vi "Sys config-process changes.vi"(11 "Initial Configuration":T1={"Triggers output setup"=[], "General trigger settings"={"Trigger 1 function"=enum."Line trigger", "Triggers loop clock (MHz)"=115.0}, "Calibration settings"={"Pockels cal.Zoom"=0, "Pockels cal.Dwell time (µs)"=0.0}, "Hardware Configuration"={"Dev. PC"=FALSE, "Swap XY on stage"=FALSE, "No of AOD"=0, "MC Supported"=FALSE, "Axial MC"=FALSE, "Computer MAC address"="", "Externalise Triggers"=FALSE, "Trigger HW config"={"Available Device List"=0, "Device Address"=""}, "DAQmx Chan"={"Pockels AO"="", "Hard shutter AO"="", "PMT AOs"="", "Galvo AOs"="", "Power meter AI"=""}, "XYZ Stage Control Config"=enum."None", "XY stage available"=FALSE, "XY Comms Config Cluster"={"Name"="", "Device Address"="", "Port "=0, "Baudrate"=0, "Comms Type"=enum."GPIB-IEEE488"}, "Y stage available"=FALSE, "Y Comms Config Cluster"={"Name"="", "Device Address"="", "Port "=0, "Baudrate"=0, "Comms Type"=enum."GPIB-IEEE488"}, "Z stage available"=FALSE, "Z Comms Config Cluster "={"Name"="", "Device Address"="", "Port "=0, "Baudrate"=0, "Comms Type"=enum."GPIB-IEEE488"}, "Encoder available"=FALSE, "Encoder"={"IP address"="224.0.1.103", "Port"=7000, "Wheel radius (cm)"=16.0, "Encoder Trigger"=""}, "VidRec available"=FALSE, "Cam VidRec"={"DO flag-Video record"="", "DO flag-Trial start"=""}, "Laser Power Control HW config"={"Laser Power Control"="", "Laser Power Modulation Control"=enum."NI"}, "Laser 1 available"=FALSE, "Laser 1 config cluster"={"COM port"="COM7", "Baud Rate"=0, "Type"=""}, "Prechirper 1 available"=FALSE, "Prechirper 1 config cluster"={"Type"="", "Baud Rate"=0, "COM port"="COM7"}, "Control system.FPGA available?"=FALSE, "Control Sys. HW config"={"Control system.FPGA Type"=enum."Virtex 5", "Control system.Network adapter name"="", "Control system.MAC address"="", "Control system.Ethernet Port"=0, "Control system.Ethernet Port Opened"=FALSE}, "DAQ FPGA HW Config"={"FGPA Ref"=refnum, "Target"="RIO0", "input card type"=enum."AC Card"}, "PMT Control Voltage Limits"={"Lower Limit"=0.0, "Upper Limit"=0.0}}, "System Config"={"Laser wavelength (nm)"=920.0, "DAQ FPGA System"={"Clock Freq (MHz) "=200.0, "Samples Wait after Trigger"=5080, "AOD fill"=4900, "StartupDelay"=0, "Slip Cycle (clock cycles)"=600000, "Add Cycle"=TRUE}, "Control system"={"AOD 1 Amplitude"=0, "AOD 2 Amplitude"=0, "AOD 3 Amplitude"=0, "AOD 4 Amplitude"=0, "AOD 5 Amplitude"=0, "AOD 6 Amplitude"=0, "T0 (ns)"=0.0, "Ta (ns)"=0.0, "Data Time Interval (ns)"=0.0, "Ctrl FPGA Clock (MHz)"=240.0}}, "Calibration config."={"Current Objective"="", "Objective Settings"=[], "PreChirper Values Preset ?"=FALSE, "PreChirper Settings"=[], "PreChirper Constants"={"a 1"=0, "b 1"=0, "c 1"=0, "a 2"=0, "b 2"=0, "c 2"=0, "lmin"=0, "lmax"=0}}, "General Setup"={"Microscope ID"="003", "Microscope Type"="AOLM", "Revision Number"="1.0.0.0", "Advanced Imaging"=FALSE, "Error Logging"=FALSE, "Performance Monitoring"=FALSE, "Max Allowed Trial Length"=60.0, "Initial Scan Resolution"=512.0, "Initial Acceptance Angle"=5.0, "Initial Laser Wavelength"=900.0, "Initial Dwell Time"=900.0}, "AOD Settings - distilled"={"AOD 1 thickness (mm)"=0.0, "AOD 2 thickness (mm)"=0.0, "AOD 3 thickness (mm)"=110.0, "AOD 4 thickness (mm)"=135.0, "AOD 1-2 separation (mm)"=15.0, "AOD 2-3 separation (mm)"=15.0, "AOD 3-4 separation (mm)"=15.0, "AOD 1 Centre (mm)"=15.0, "AOD 2 Centre (mm)"=50.0, "AOD 3 Centre (mm)"=50.0, "AOD 4 Centre (mm)"=50.0, "AOD 1 X Offset"=15.0, "AOD 2 X Offset"=1.0, "AOD 3 X Offset"=1.0, "AOD 4 X Offset"=1.0, "AOD 1 Y Offset"=1.0, "AOD 2 Y Offset"=1.0, "AOD 3 Y Offset"=1.0, "AOD 4 Y Offset"=1.0, "Timing Offset AOD 1"=0.0, "Timing Offset AOD 2"=0.0, "Timing Offset AOD 3"=0.0, "Timing Offset AOD 4"=0.0, "AOL centre wavelength (nm)"=1.0, "AOL centre frequency (MHz)"=1.0, "Pair deflection ratio"=1.0, "AOL aperture (mm)"=0.0, "AOD fill time (us)"=0.0, "Diffraction mode"=0.0, "Crystal length (mm)"=0.0, "Acoustic velocity (m/s)"=1.0, "AOD Ord. Refractive index"=20000.0}} {"System Config"."Control system"."Ctrl FPGA Clock (MHz)" min=80.0 max=500.0 step=1.0; "System Config"."Control system"."Data Time Interval (ns)" min=0.0 max=2048.0 step=1.0; "System Config"."Control system"."Ta (ns)" min=0.0 max=2048.0 step=1.0; "System Config"."Control system"."T0 (ns)" min=0.0 max=2048.0 step=1.0; "System Config"."Control system"."AOD 6 Amplitude" min=0 max=2048 step=1; "System Config"."Control system"."AOD 5 Amplitude" min=0 max=2048 step=1; "System Config"."Control system"."AOD 4 Amplitude" min=0 max=2048 step=1; "System Config"."Control system"."AOD 3 Amplitude" min=0 max=2048 step=1; "System Config"."Control system"."AOD 2 Amplitude" min=0 max=2048 step=1; "System Config"."Control system"."AOD 1 Amplitude" min=0 max=2048 step=1; "System Config"."Laser wavelength (nm)" min=800.0 max=1080.0 step=1.0; "Hardware Configuration"."Encoder"."Wheel radius (cm)" format="%#_13g"; "General trigger settings"."Triggers loop clock (MHz)" format="%#_13g"; "Triggers output setup"."Pulse width (us)" min=10 max=5000 step=1 format="%.0fµs"}) -> ()   [LabVIEW 2020]
uses:
  Visualisation/Functional Imaging Viewer/Typedefs/Get-Set-Clear Control.ctl
  Typedefs/HW config states enum.ctl
  Typedefs/Save-Load enum.ctl
  Peripherals Control/Triggers/Typedefs/Trigger setup element cluster.ctl
  Peripherals Control/Triggers/Typedefs/Triggers output setup.ctl
  Configuration code/Typedefs/Pockels Calibration settings cluster.ctl
  Typedefs/Trigger 1 selector enum.ctl
  Peripherals Control/Triggers/Typedefs/General trigger settings cluster.ctl
  Typedefs/Cam VidRec HW config setup cluster.ctl
  Typedefs/Control Sys HW config cluster.ctl
  <vilib>/userDefined/High Color/nirio_resource_hc.ctl
  Typedefs/FPGA input type AC-DC.ctl
  RIG-SPECIFIC FILES/FPGA Refs/FPGA Ref.ctl
  Typedefs/DAQ FPGA HW config cluster.ctl
  Typedefs/DAQmx physical channels cluster.ctl
  Typedefs/Encoder config cluster.ctl
  Typedefs/Laser 1 config cluster.ctl
  Typedefs/PreChirper 1 config cluster.ctl
  Typedefs/Laser Power Control HW config.ctl
  Typedefs/Triggers HW config.ctl
  Typedefs/Hardware Configuration settings.ctl
  Typedefs/DAQ FPGA system config.ctl
  Typedefs/CTRL system config.ctl
  Typedefs/System Configuration.ctl
  Typedefs/Objective Config.ctl
  Typedefs/Prechirper Cal Config.ctl
  Typedefs/PreChirper constants.ctl
  Typedefs/Calibration config.ctl
  Typedefs/General Setup.ctl
  Typedefs/AOD Settings-distilled.ctl
  Configuration code/Typedefs/Initial config.ctl
  Typedefs/PMT Control Voltage limits.ctl
  Peripherals Control/XYZ Stage/Control/typedefs/XYZControlConfig.ctl
  Typedefs/Comms Type.ctl
  Typedefs/Peripherals comms config cluster.ctl
panel:
  # "Thickness (mm)"
  # "X Offset"
  # "Separation (mm)"
  # "Y Offset"
  # "Centre (mm)"
  # "Timing Offset"
  # "(make , model etc)"
  # "(COM Port / IP Address / service address etc.)"
  # "(Port for ethernet / channel for BT)"
  # "(make , model etc)"
  # "(COM Port / IP Address / service address etc.)"
  # "(Port for ethernet / channel for BT)"
  # "(make , model etc)"
  # "(COM Port / IP Address / service address etc.)"
  # "(Port for ethernet / channel for BT)"
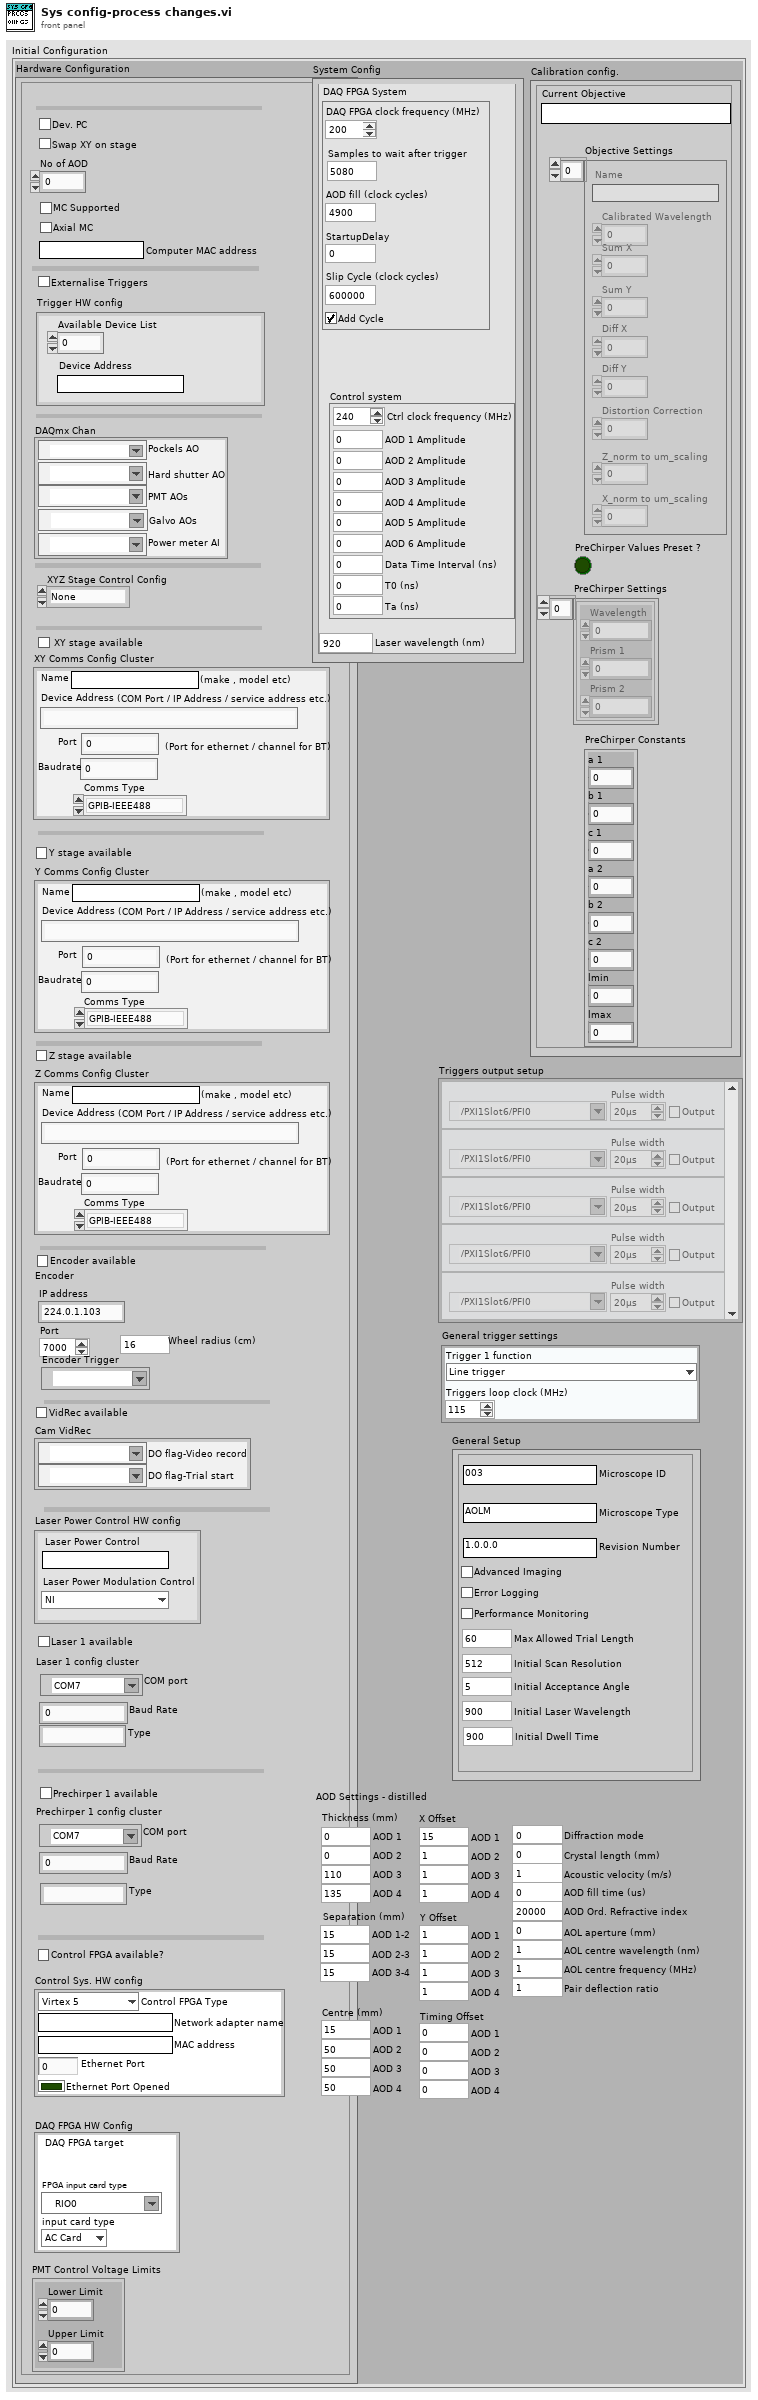
[diagram p1: front panel]
types:
  T1 = typedef "Initial config.ctl" = cluster{"Triggers output setup":T2, "General trigger settings":T4, "Calibration settings":T6, "Hardware Configuration":T7, "System Config":T24, "Calibration config.":T27, "General Setup":T31, "AOD Settings - distilled":T32}
  T2 = typedef "Triggers output setup.ctl" = T3[]
  T3 = typedef "Trigger setup element cluster.ctl" = cluster{"Name":string, "Output?":bool, "Output terminal":tag, "PXI backplane line":tag, "Pulse width (us)":u16}
  T4 = typedef "General trigger settings cluster.ctl" = cluster{"Trigger 1 function":T5, "Triggers loop clock (MHz)":dbl}
  T5 = typedef "Trigger 1 selector enum.ctl" = enum16{"Encoder trigger", "Line trigger", "Control system's ref frame acknowledgement"}
  T6 = typedef "Pockels Calibration settings cluster.ctl" = cluster{"Pockels cal.Zoom":u8, "Pockels cal.Dwell time (µs)":dbl}
  T7 = typedef "Hardware Configuration settings.ctl" = cluster{"Dev. PC":bool, "Swap XY on stage":bool, "No of AOD":u8, "MC Supported":bool, "Axial MC":bool, "Computer MAC address":string, "Externalise Triggers":bool, "Trigger HW config":T8, "DAQmx Chan":T9, "XYZ Stage Control Config":T10, "XY stage available":bool, "XY Comms Config Cluster":T11, "Y stage available":bool, "Y Comms Config Cluster":T11, "Z stage available":bool, "Z Comms Config Cluster ":T11, "Encoder available":bool, "Encoder":T13, "VidRec available":bool, "Cam VidRec":T14, "Laser Power Control HW config":T15, "Laser 1 available":bool, "Laser 1 config cluster":T16, "Prechirper 1 available":bool, "Prechirper 1 config cluster":T17, "Control system.FPGA available?":bool, "Control Sys. HW config":T18, "DAQ FPGA HW Config":T19, "PMT Control Voltage Limits":T23}
  T8 = typedef "Triggers HW config.ctl" = cluster{"Available Device List":i32, "Device Address":string}
  T9 = typedef "DAQmx physical channels cluster.ctl" = cluster{"Pockels AO":tag, "Hard shutter AO":tag, "PMT AOs":tag, "Galvo AOs":tag, "Power meter AI":tag}
  T10 = typedef "XYZControlConfig.ctl" = enum16{"None", "XYZ", "XY-Z", "X-Y-Z", "Z"}
  T11 = typedef "Peripherals comms config cluster.ctl" = cluster{"Name":string, "Device Address":string, "Port ":u16, "Baudrate":i32, "Comms Type":T12}
  T12 = typedef "Comms Type.ctl" = enum16{"GPIB-IEEE488", "Serial-RS232", "Serial-RS485", "Serial-RS422", "Serial-USB", "Ethernet-TCP/IP", "Ethernet-UDP"}
  T13 = typedef "Encoder config cluster.ctl" = cluster{"IP address":string, "Port":u16, "Wheel radius (cm)":dbl, "Encoder Trigger":tag}
  T14 = typedef "Cam VidRec HW config setup cluster.ctl" = cluster{"DO flag-Video record":tag, "DO flag-Trial start":tag}
  T15 = typedef "Laser Power Control HW config.ctl" = cluster{"Laser Power Control":string, "Laser Power Modulation Control":enum16{"NI", "FPGA"}}
  T16 = typedef "Laser 1 config cluster.ctl" = cluster{"COM port":refnum<visa-resource-name>, "Baud Rate":i32, "Type":string}
  T17 = typedef "PreChirper 1 config cluster.ctl" = cluster{"Type":string, "Baud Rate":i32, "COM port":refnum<visa-resource-name>}
  T18 = typedef "Control Sys HW config cluster.ctl" = cluster{"Control system.FPGA Type":enum16{"Virtex 5", "Virtex 7"}, "Control system.Network adapter name":string, "Control system.MAC address":string, "Control system.Ethernet Port":u32, "Control system.Ethernet Port Opened":bool}
  T19 = typedef "DAQ FPGA HW config cluster.ctl" = cluster{"FGPA Ref":T20, "Target":T21, "input card type":T22}
  T20 = typedef "FPGA Ref.ctl" = refnum<k20>
  T21 = typedef "nirio_resource_hc.ctl" = tag
  T22 = typedef "FPGA input type AC-DC.ctl" = enum16{"AC Card", "DC Card"}
  T23 = typedef "PMT Control Voltage limits.ctl" = cluster{"Lower Limit":dbl, "Upper Limit":dbl}
  T24 = typedef "System Configuration.ctl" = cluster{"Laser wavelength (nm)":dbl, "DAQ FPGA System":T25, "Control system":T26}
  T25 = typedef "DAQ FPGA system config.ctl" = cluster{"Clock Freq (MHz) ":dbl, "Samples Wait after Trigger":u16, "AOD fill":u16, "StartupDelay":i32, "Slip Cycle (clock cycles)":u32, "Add Cycle":bool}
  T26 = typedef "CTRL system config.ctl" = cluster{"AOD 1 Amplitude":i16, "AOD 2 Amplitude":i16, "AOD 3 Amplitude":i16, "AOD 4 Amplitude":i16, "AOD 5 Amplitude":i16, "AOD 6 Amplitude":i16, "T0 (ns)":dbl, "Ta (ns)":dbl, "Data Time Interval (ns)":dbl, "Ctrl FPGA Clock (MHz)":dbl}
  T27 = typedef "Calibration config.ctl" = cluster{"Current Objective":string, "Objective Settings":T28[], "PreChirper Values Preset ?":bool, "PreChirper Settings":T29[], "PreChirper Constants":T30}
  T28 = typedef "Objective Config.ctl" = cluster{"Name":string, "Sum X":dbl, "Sum Y":dbl, "Diff X":dbl, "Diff Y":dbl, "Distortion Correction":dbl, "Z_norm to um_scaling":dbl, "X_norm to um_scaling":dbl, "Calibrated Wavelength":dbl}
  T29 = typedef "Prechirper Cal Config.ctl" = cluster{"Wavelength":i32, "Prism 1":i32, "Prism 2":i32}
  T30 = typedef "PreChirper constants.ctl" = cluster{"a 1":i32, "b 1":i32, "c 1":i32, "a 2":i32, "b 2":i32, "c 2":i32, "lmin":i32, "lmax":i32}
  T31 = typedef "General Setup.ctl" = cluster{"Microscope ID":string, "Microscope Type":string, "Revision Number":string, "Advanced Imaging":bool, "Error Logging":bool, "Performance Monitoring":bool, "Max Allowed Trial Length":dbl, "Initial Scan Resolution":dbl, "Initial Acceptance Angle":dbl, "Initial Laser Wavelength":dbl, "Initial Dwell Time":dbl}
  T32 = typedef "AOD Settings-distilled.ctl" = cluster{"AOD 1 thickness (mm)":dbl, "AOD 2 thickness (mm)":dbl, "AOD 3 thickness (mm)":dbl, "AOD 4 thickness (mm)":dbl, "AOD 1-2 separation (mm)":dbl, "AOD 2-3 separation (mm)":dbl, "AOD 3-4 separation (mm)":dbl, "AOD 1 Centre (mm)":dbl, "AOD 2 Centre (mm)":dbl, "AOD 3 Centre (mm)":dbl, "AOD 4 Centre (mm)":dbl, "AOD 1 X Offset":dbl, "AOD 2 X Offset":dbl, "AOD 3 X Offset":dbl, "AOD 4 X Offset":dbl, "AOD 1 Y Offset":dbl, "AOD 2 Y Offset":dbl, "AOD 3 Y Offset":dbl, "AOD 4 Y Offset":dbl, "Timing Offset AOD 1":dbl, "Timing Offset AOD 2":dbl, "Timing Offset AOD 3":dbl, "Timing Offset AOD 4":dbl, "AOL centre wavelength (nm)":dbl, "AOL centre frequency (MHz)":dbl, "Pair deflection ratio":dbl, "AOL aperture (mm)":dbl, "AOD fill time (us)":dbl, "Diffraction mode":dbl, "Crystal length (mm)":dbl, "Acoustic velocity (m/s)":dbl, "AOD Ord. Refractive index":dbl}
  T33 = typedef "Get-Set-Clear Control.ctl" = enum16{"Get", "Set", "Clear"}
  T34 = typedef "HW config states enum.ctl" = enum16{"Load from file", "Save to file", "Save backup", "Write all", "Read all", "Write XY stage settings", "Write DAQ FPGA settings", "Write Control FPGA settings", "Write Phys Channels", "Write System Config", "Write HW Config", "Save System Config", "Save HW Config", "Clear", "Compare from file"}
  T35 = enum16{"Initialise", "Load from file", "Save to file", "Read", "Write"}
  T36 = typedef "Save-Load enum.ctl" = enum16{"Save to file", "Load from file", "Compare from file", "Save Backup"}
  T37 = typedef "AOL Properties Cluster.ctl" = cluster{"AOD 1 thickness (mm)":dbl, "AOD 2 thickness (mm)":dbl, "AOD 3 thickness (mm)":dbl, "AOD 4 thickness (mm)":dbl, "AOD 5 thickness (mm)":dbl, "AOD 6 thickness (mm)":dbl, "AOD 1-2 separation (mm)":dbl, "AOD 2-3 separation (mm)":dbl, "AOD 3-4 separation (mm)":dbl, "AOD 4-5 separation (mm)":dbl, "AOD 5-6 separation (mm)":dbl, "AOD 1 X Offset":dbl, "AOD 2 X Offset":dbl, "AOD 3 X Offset":dbl, "AOD 4 X Offset":dbl, "AOD 1 Y Offset":dbl, "AOD 2 Y Offset":dbl, "AOD 3 Y Offset":dbl, "AOD 4 Y Offset":dbl, "AOD 1 X Direction":dbl, "AOD 2 X Direction":dbl, "AOD 3 X Direction":dbl, "AOD 4 X Direction":dbl, "AOD 1 Y Direction":dbl, "AOD 2 Y Direction":dbl, "AOD 3 Y Direction":dbl, "AOD 4 Y Direction":dbl, "AOD 1 Centre (mm)":dbl, "AOD 2 Centre (mm)":dbl, "AOD 3 Centre (mm)":dbl, "AOD 4 Centre (mm)":dbl, "Timing Offset AOD 1":dbl, "Timing Offset AOD 2":dbl, "Timing Offset AOD 3":dbl, "Timing Offset AOD 4":dbl, "AOD Optical offset 1":dbl, "AOD Optical offset 2":dbl, "AOL aperture (mm)":dbl, "AOL centre wavelength (nm)":dbl, "AOL centre frequency (MHz)":dbl, "Diffraction mode":dbl, "Crystal length (mm)":dbl, "Acoustic velocity (m/s)":dbl, "Pair deflection ratio":dbl, "AOD fill time (us)":dbl, "AOD Ord. Refractive index":dbl, "AOD ExtraOrd. Refractive index":dbl}
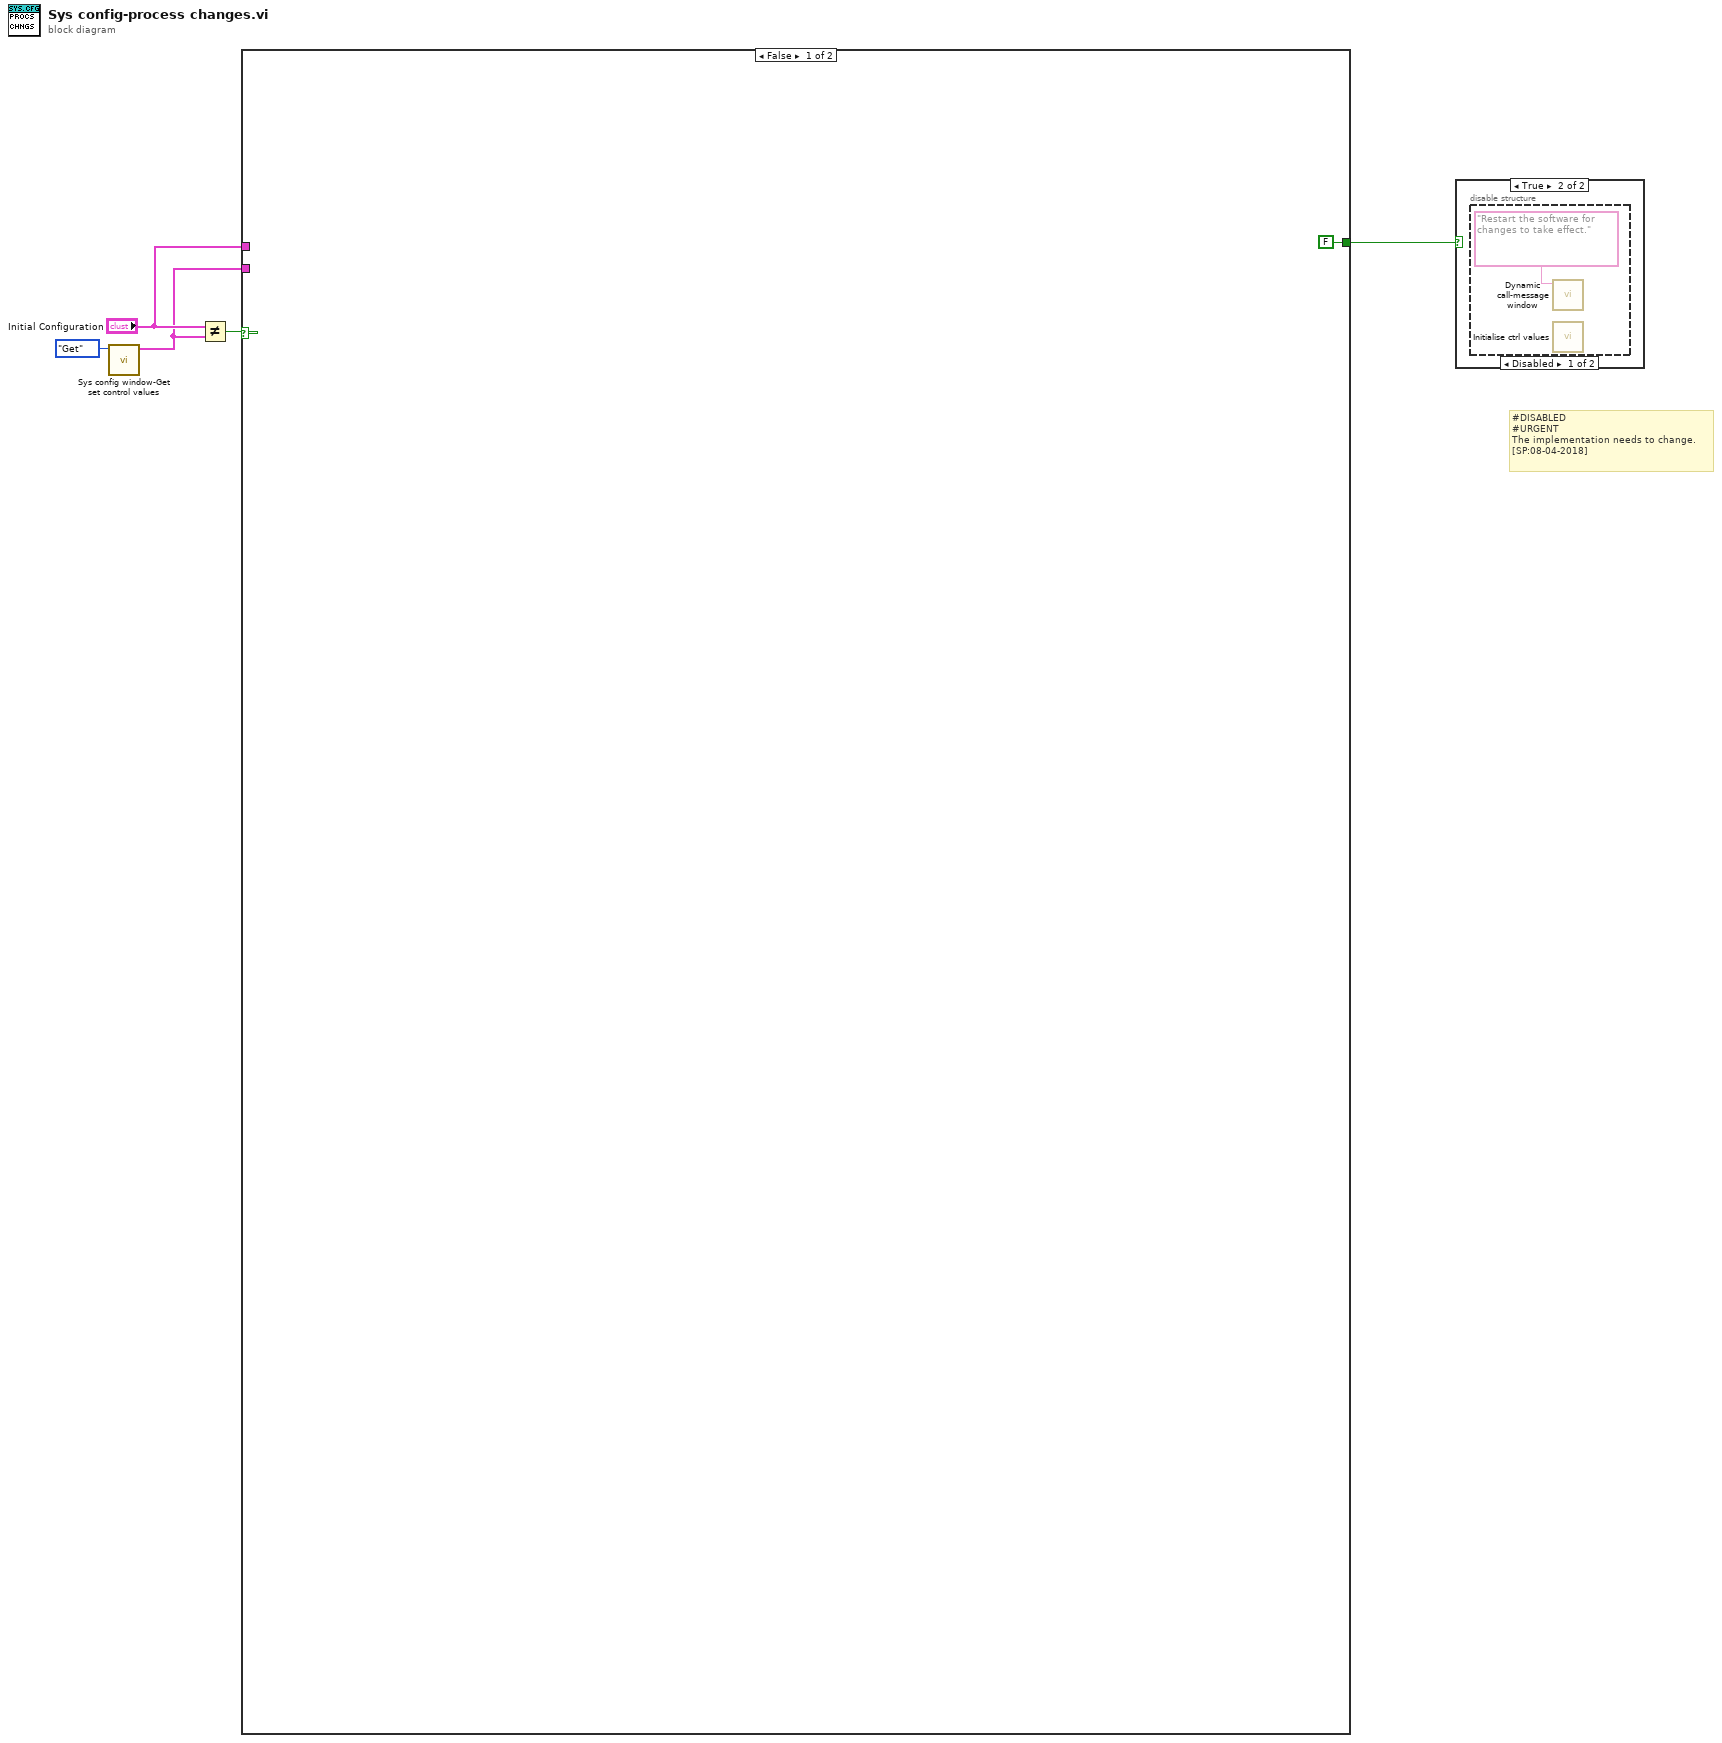
[diagram p0: block diagram]
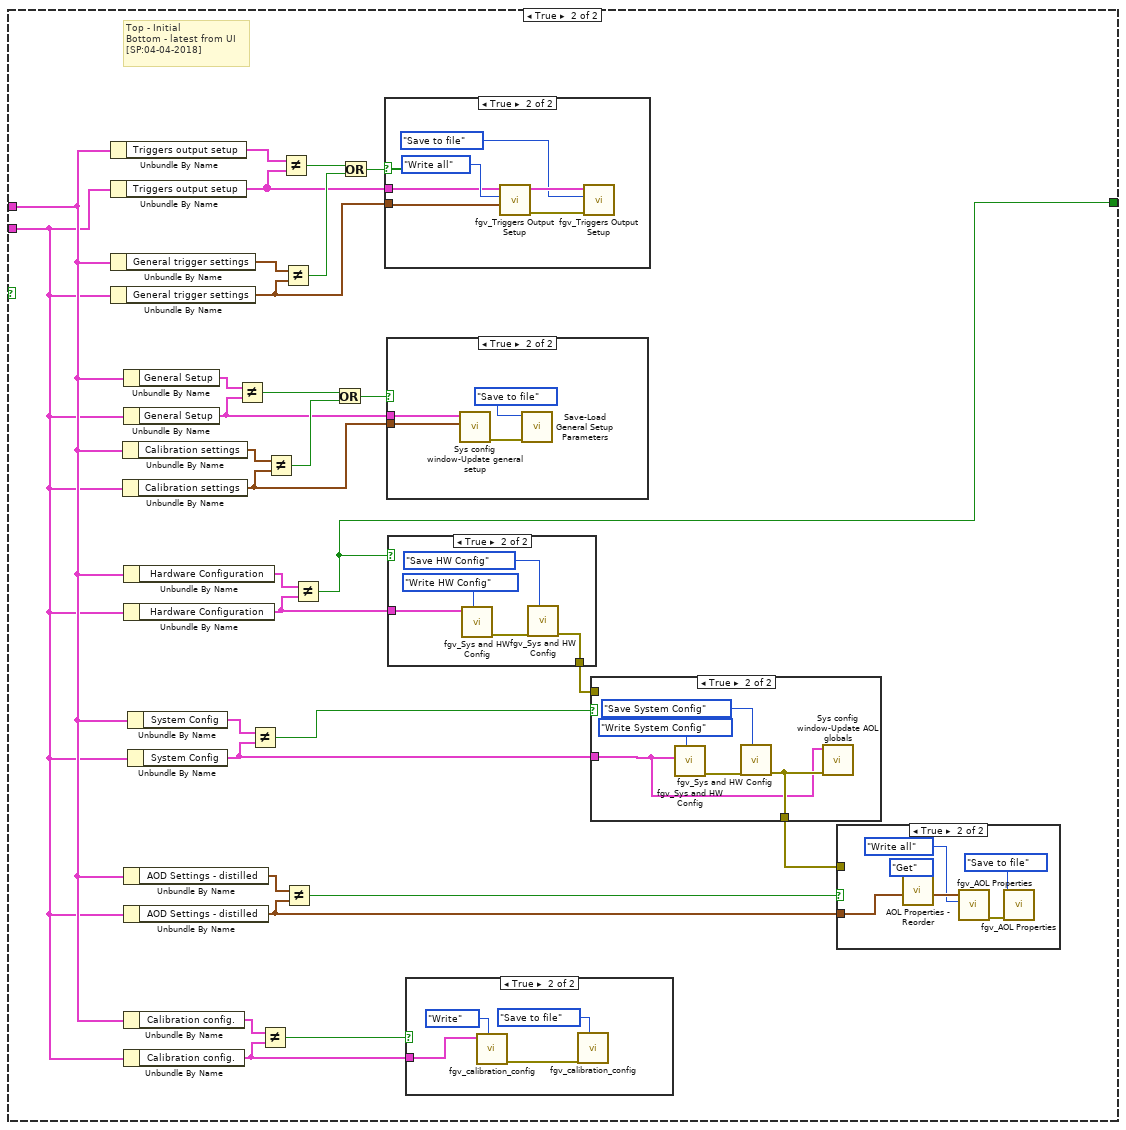
[diagram p4: hidden frame]
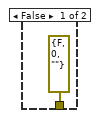
[diagram p6: hidden frame]
diagram:
  # "#DISABLED\n#URGENT\nThe implementation needs to change.\n[SP:08-04-2018]"
  n1 = call "Sys config window-Get set control values.vi"("Function"=Get-Set-Clear_Control."Get") -> ("output cluster"=w2:T1)  [unwired: 9 in, 1 out]
  n2 = Not Equal?(x="Initial Configuration", y=w2) -> (x != y?=w4:bool)
  n3 = case shown="False" w4 {
    tunnel: "Initial Configuration" -> [_ w36]
    tunnel: w2 -> [_ w35]
    tunnel: [FALSE w7] -> w1
    frame False {
    }
    frame True {
      # "Top - Initial\nBottom - latest from UI\n[SP:04-04-2018]"
      n4 = Unbundle By Name(w36) -> ("Triggers output setup"=w34:T2)
      n5 = Unbundle By Name(w35) -> ("Triggers output setup"=w23:T2)
      n6 = Unbundle By Name(w36) -> ("General trigger settings"=w33:T4)
      n7 = Unbundle By Name(w35) -> ("General trigger settings"=w22:T4)
      n8 = Unbundle By Name(w36) -> ("Calibration settings"=w32:T6)
      n9 = Unbundle By Name(w35) -> ("Calibration settings"=w14:T6)
      n10 = Unbundle By Name(w36) -> ("General Setup"=w28:T31)
      n11 = Unbundle By Name(w35) -> ("General Setup"=w15:T31)
      n12 = Unbundle By Name(w36) -> ("Hardware Configuration"=w31:T7)
      n13 = Unbundle By Name(w35) -> ("Hardware Configuration"=w13:T7)
      n14 = Unbundle By Name(w36) -> ("AOD Settings - distilled"=w27:T32)
      n15 = Unbundle By Name(w35) -> ("AOD Settings - distilled"=w8:T32)
      n16 = Unbundle By Name(w36) -> ("Calibration config."=w29:T27)
      n17 = Unbundle By Name(w35) -> ("Calibration config."=w16:T27)
      n18 = Unbundle By Name(w36) -> ("System Config"=w30:T24)
      n19 = Unbundle By Name(w35) -> ("System Config"=w11:T24)
      n20 = Not Equal?(x=w28, y=w15) -> (x != y?=w21:bool)
      n21 = Not Equal?(x=w30, y=w11) -> (x != y?=w12:bool)
      n22 = Not Equal?(x=w29, y=w16) -> (x != y?=w18:bool)
      n23 = Not Equal?(x=w32, y=w14) -> (x != y?=w20:bool)
      n24 = Not Equal?(x=w34, y=w23) -> (x != y?=w26:bool)
      n25 = Not Equal?(x=w33, y=w22) -> (x != y?=w25:bool)
      n26 = Not Equal?(x=w27, y=w8) -> (x != y?=w17:bool)
      n27 = Not Equal?(x=w31, y=w13) -> (x != y?=w7:bool)
      n28 = Or(x=w21, y=w20) -> (x .or. y?=w19:bool)
      n29 = Or(x=w26, y=w25) -> (x .or. y?=w24:bool)
      n30 = case shown="True" w24 {
        tunnel: w23 -> [_ w67]
        tunnel: w22 -> [_ w66]
        frame False {
        }
        frame True {
          n31 = call "fgv_Triggers Output Setup.vi"("General trigger settings"=w66, "Function"=HW_config_states_enum."Write all", "Triggers output setup"=w67) -> ("error out"=w65:errorcluster, "Triggers output setup"=w64:T2)  [unwired: 6 in, 1 out]
          n32 = call "fgv_Triggers Output Setup.vi"("error in (no error)"=w65, "Function"=HW_config_states_enum."Save to file", "Triggers output setup"=w64) -> ()  [unwired: 6 in, 3 out]
        }
      }
      n33 = case shown="True" w19 {
        tunnel: w15 -> [_ w60]
        tunnel: w14 -> [_ w61]
        frame False {
        }
        frame True {
          n34 = call "Sys config window-Update general setup.vi"("Calibration settings"=w61, "General Setup"=w60) -> ("error out"=w59:errorcluster)  [unwired: 9 in]
          n35 = call "Save-Load General Setup Parameters.vi"("error in"=w59, "Function"=Save-Load_enum."Save to file") -> ()  [unwired: 9 in, 1 out]
        }
      }
      n36 = case shown="True" w7 {
        tunnel: w13 -> [_ w47]
        tunnel: [errorcluster {"status"=FALSE, "code"=0, "source"=""} ("error out") w44] -> w10
        frame False {
        }
        frame True {
          n37 = call "fgv_Sys and HW Config.vi"("Function"=HW_config_states_enum."Write HW Config", "Hardware Configuration"=w47) -> ("error out"=w45:errorcluster)  [unwired: 7 in, 2 out]
          n38 = call "fgv_Sys and HW Config.vi"("Function"=HW_config_states_enum."Save HW Config", "error in (no error)"=w45) -> ("error out"=w44:errorcluster)  [unwired: 7 in, 2 out]
        }
      }
      n39 = case shown="True" w18 {
        tunnel: w16 -> [_ w57]
        frame False {
        }
        frame True {
          n40 = call "fgv_calibration_config.vi"("Cal config ops"=T35."Write", "Config cluster IN"=w57) -> ("error out"=w55:errorcluster)  [unwired: 7 in, 2 out]
          n41 = call "fgv_calibration_config.vi"("Cal config ops"=T35."Save to file", "error in (no error)"=w55) -> ()  [unwired: 7 in, 3 out]
        }
      }
      n42 = case shown="True" w12 {
        tunnel: w11 -> [_ w38]
        tunnel: w10 -> [w37 _]
        tunnel: [w37 w39] -> w9
        frame False {
        }
        frame True {
          n43 = call "fgv_Sys and HW Config.vi"("Function"=HW_config_states_enum."Write System Config", "System Config"=w38) -> ("error out"=w42:errorcluster)  [unwired: 7 in, 2 out]
          n44 = call "fgv_Sys and HW Config.vi"("Function"=HW_config_states_enum."Save System Config", "error in (no error)"=w42) -> ("error out"=w39:errorcluster)  [unwired: 7 in, 2 out]
          n45 = call "Sys config window-Update AOL globals.vi"("error in (no error)"=w39, "System Config"=w38) -> ()  [unwired: 9 in, 1 out]
        }
      }
      n46 = case shown="True" w17 {
        tunnel: w9 -> [_ _]
        tunnel: w8 -> [_ w52]
        frame False {
        }
        frame True {
          n47 = call "AOL Properties - Reorder.vi"("Function"=Get-Set-Clear_Control."Get", "Value"=w52) -> ("AOL Properties out"=w53:T37)  [unwired: 8 in, 1 out]
          n48 = call "fgv_AOL Properties.vi"("Function"=HW_config_states_enum."Write all", "AOL Properties in"=w53) -> ("error out"=w50:errorcluster)  [unwired: 8 in, 1 out]
          n49 = call "fgv_AOL Properties.vi"("error in (no error)"=w50, "Function"=HW_config_states_enum."Save to file") -> ()  [unwired: 8 in, 2 out]
        }
      }
    }
  }
  n50 = case shown="True" w1 {
    frame False {
    }
    frame True {
      n51 = disable-structure shown="Disabled" {
        frame Disabled {
          n52 = call "Dynamic call-message window.vi"("Message"="Restart the software for changes to take effect.") -> ()  [unwired: 10 in, 1 out]
          n53 = call "Initialise ctrl values.vi"() -> ()  [unwired: 11 in, 1 out]
        }
        frame Enabled {
        }
      }
    }
  }
